vi "Move Conveyer Belt.vi"(7 "Enable Stack":bool, 8 "frisbee counter":i16, 9 "Suck":bool) -> (0 "move conveyer belt":bool)   [LabVIEW 2012]
uses:
  BotStatus.vi
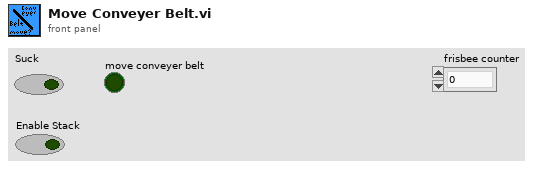
[diagram p1: front panel]
types:
  T1 = cluster{"Middle":bool, "InCannon":bool, "InFlipper":bool, "Bottom":bool, "FlipperDown":bool}
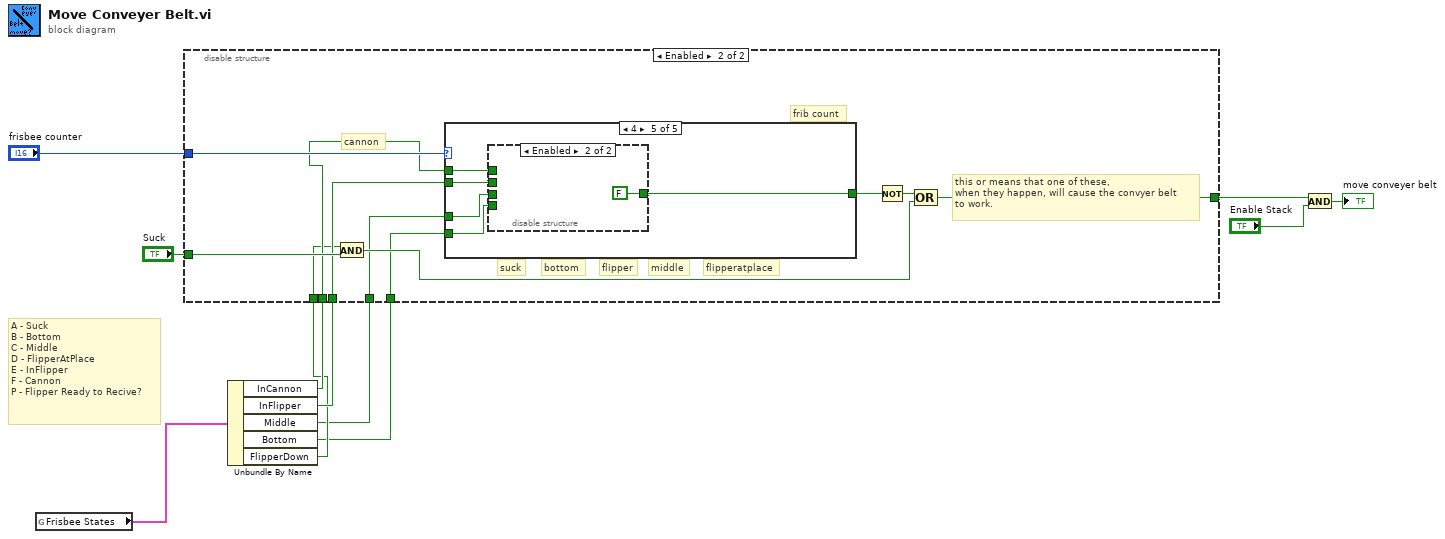
[diagram p0: block diagram]
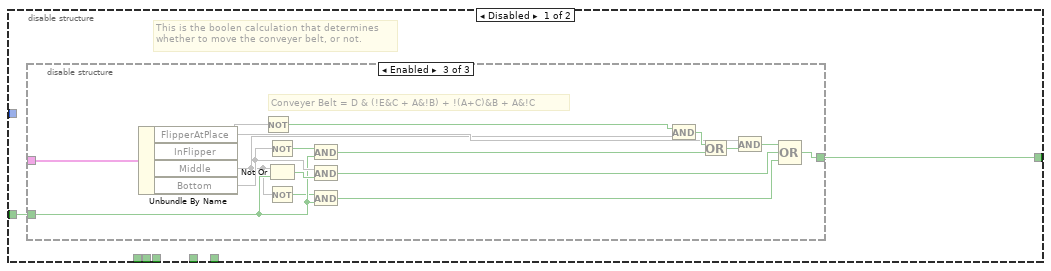
[diagram p2: hidden frame]
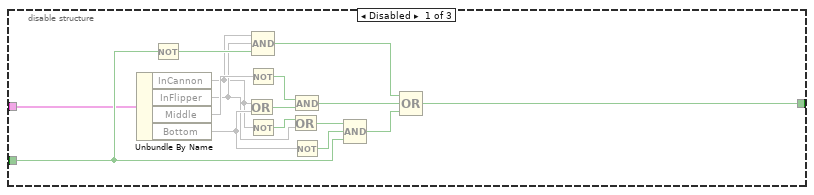
[diagram p3: hidden frame]
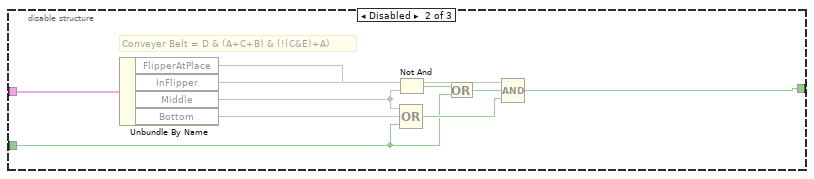
[diagram p4: hidden frame]
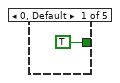
[diagram p5: hidden frame]
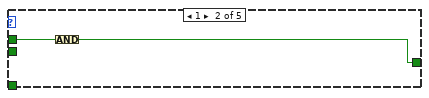
[diagram p6: hidden frame]
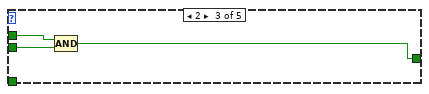
[diagram p7: hidden frame]
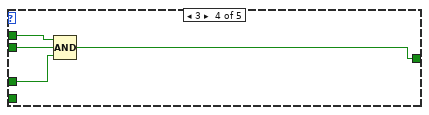
[diagram p8: hidden frame]
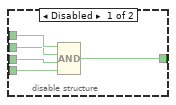
[diagram p9: hidden frame]
diagram:
  # "A - Suck\nB - Bottom\nC - Middle\nD - FlipperAtPlace\nE - InFlipper\nF - Cannon\nP - Flipper Ready to Recive?"
  n1 = global read "BotStatus.vi" "Frisbee States"() -> (w6:T1)
  n2 = Unbundle By Name(w6) -> ("InCannon"=w5:bool, "InFlipper"=w4:bool, "Middle"=w2:bool, "Bottom"=w1:bool, "FlipperDown"=w3:bool)
  n3 = disable-structure shown="Enabled" {
    disable-tunnel: "Suck" -> [w13 w63]
    disable-tunnel: "frisbee counter" -> [_ w65]
    disable-tunnel: [w12 w64] -> w7
    disable-tunnel: w5 -> [_ w61]
    disable-tunnel: w4 -> [_ w60]
    disable-tunnel: w3 -> [_ w59]
    disable-tunnel: w2 -> [_ w58]
    disable-tunnel: w1 -> [_ w57]
    frame Disabled {
      # "This is the boolen calculation that determines\nwhether to move the conveyer belt, or not."
      n4 = disable-structure shown="Enabled" {
        disable-tunnel: [w16 w37 w40] -> w12
        disable-tunnel: w13 -> [w15 w31 w44]
        disable-tunnel: _ -> [w14 w39 w56]
        frame Disabled {
          n5 = Unbundle By Name(w14) -> ("InCannon"=w18, "InFlipper"=w19, "Middle"=w26, "Bottom"=w23)
          n6 = Not(x=w15) -> (.not. x?=w20:bool)
          n7 = Or(x=w18, y=w23) -> (x .or. y?=w24:bool)
          n8 = Not(x=w26) -> (.not. x?=w25:bool)
          n9 = Not(x=w18) -> (.not. x?=w28:bool)
          n10 = Compound Arithmetic op=AND(w18, w19, w20) -> (w17:bool)
          n11 = Or(x=w28, y=w19) -> (x .or. y?=w27:bool)
          n12 = And(x=w25, y=w24) -> (x .and. y?=w22:bool)
          n13 = Not(x=w23) -> (.not. x?=w29:bool)
          n14 = Compound Arithmetic op=AND(w27, w29, w15) -> (w21:bool)
          n15 = Compound Arithmetic op=OR(w17, w22, w21) -> (w16:bool)
        }
        frame Disabled {
          # "Conveyer Belt = D & (A+C+B) & (!(C&E)+A)"
          n16 = Unbundle By Name(w39) -> ("FlipperAtPlace"=w36, "InFlipper"=w34, "Middle"=w33, "Bottom"=w38)
          n17 = Not And(1:w33, 2:w34) -> (0:w32:bool)
          n18 = Compound Arithmetic op=OR(w33, w38, w31) -> (w35:bool)
          n19 = Or(x=w32, y=w31) -> (x .or. y?=w30:bool)
          n20 = Compound Arithmetic op=AND(w36, w30, w35) -> (w37:bool)
        }
        frame Enabled {
          # "Conveyer Belt = D & (!E&C + A&!B) + !(A+C)&B + A&!C"
          n21 = Unbundle By Name(w56) -> ("FlipperAtPlace"=w49, "InFlipper"=w55, "Middle"=w42, "Bottom"=w46)
          n22 = Not(x=w55) -> (.not. x?=w54:bool)
          n23 = Not(x=w46) -> (.not. x?=w51:bool)
          n24 = Not Or(1:w44, 2:w42) -> (0:w47:bool)
          n25 = Not(x=w42) -> (.not. x?=w43:bool)
          n26 = And(x=w51, y=w44) -> (x .and. y?=w52:bool)
          n27 = And(x=w46, y=w47) -> (x .and. y?=w45:bool)
          n28 = And(x=w43, y=w44) -> (x .and. y?=w41:bool)
          n29 = And(x=w54, y=w42) -> (x .and. y?=w53:bool)
          n30 = Or(x=w53, y=w52) -> (x .or. y?=w50:bool)
          n31 = And(x=w49, y=w50) -> (x .and. y?=w48:bool)
          n32 = Compound Arithmetic op=OR(w48, w45, w41) -> (w40:bool)
        }
      }
    }
    frame Enabled {
      # "bottom"
      # "middle"
      # "flipperatplace"
      # "flipper"
      # "cannon"
      # "frib count"
      # "suck"
      # "this or means that one of these, \nwhen they happen, will cause the convyer belt\nto work."
      n33 = And(x=w59, y=w63) -> (x .and. y?=w62:bool)
      n34 = case shown="4" w65 {
        tunnel: w61 -> [_ w70 w72 w76 w82]
        tunnel: w60 -> [_ _ w73 w77 w81]
        tunnel: [TRUE w69 w71 w75 w78] -> w66
        tunnel: w58 -> [_ _ _ w74 w80]
        tunnel: w57 -> [_ _ _ _ w79]
        frame 0, Default {
        }
        frame 1 {
          n35 = Compound Arithmetic op=AND(w70) -> (w69:bool)
        }
        frame 2 {
          n36 = Compound Arithmetic op=AND(w72, w73) -> (w71:bool)
        }
        frame 3 {
          n37 = Compound Arithmetic op=AND(w76, w77, w74) -> (w75:bool)
        }
        frame 4 {
          n38 = disable-structure shown="Enabled" {
            disable-tunnel: w82 -> [w87 _]
            disable-tunnel: w81 -> [w86 _]
            disable-tunnel: w80 -> [w85 _]
            disable-tunnel: w79 -> [w84 _]
            disable-tunnel: [w83 FALSE] -> w78
            frame Disabled {
              n39 = Compound Arithmetic op=AND(w87, w86, w85, w84) -> (w83:bool)
            }
            frame Enabled {
            }
          }
        }
      }
      n40 = Not(x=w66) -> (.not. x?=w67:bool)
      n41 = Compound Arithmetic op=OR(w67, w62) -> (w64:bool)
    }
  }
  n42 = And(x=w7, y="Enable Stack") -> (x .and. y?=→"move conveyer belt":bool)
